vi "Stop.vi"(8 "error in (no error)":errorcluster, 10 "Message in":refnum<class "StopMessage.lvclass">, 11 "DAQCascade512II in":refnum<class "DAQCascade512II.lvclass">) -> (0 "error out":errorcluster, 3 "DAQCascade512II out":refnum<class "DAQCascade512II.lvclass">)   [LabVIEW 2012, in "DAQCascade512II.lvclass"]
doc: "This member function is called when the statemachine in the run.vi receives an 'stop' command. It relays the message to all observers of the component.\n\nOverride this member function in your derived class if you need additional stop functionality (but don't forget to call the parent method)."
uses:
  DAQCascade512II.lvclass
  <vilib>/Distrio/Murmex/StopMessage/StopMessage.lvclass
  <vilib>/Distrio/Murmex/Murmex/Murmex.lvclass
  DAQCascade512II.lvclass/DAQCascade512II.ctl
  <vilib>/Distrio/Murmex/TerminateMessage/TerminateMessage class.ctl
  <vilib>/Distrio/Murmex/TerminateMessage/TerminateMessage.lvclass
panel:
  # "This method is called when the STOP\ntrigger is sent. \n\nOverride this method when your component needs to\nrespond to this trigger. \n\nCall parent for proper implementation"
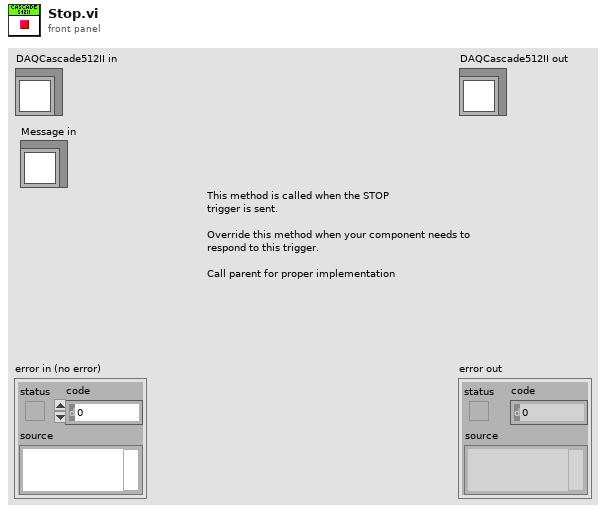
[diagram p1: front panel]
types:
  T1 = typedef "Murmex.lvlib/TerminateMessage.lvclass/TerminateMessage class.ctl" = refnum<class "TerminateMessage.lvclass">
  T2 = typedef "IMAQ Image.ctl" = refnum<image>
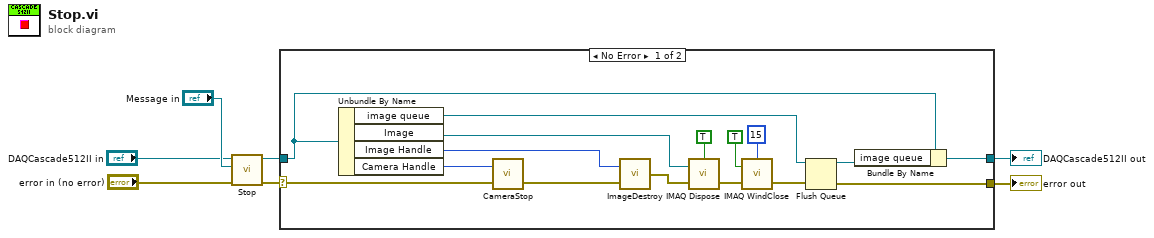
[diagram p0: block diagram]
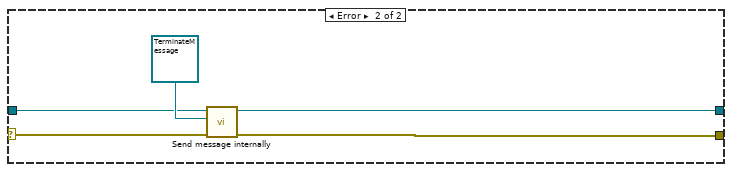
[diagram p2: hidden frame]
diagram:
  n1 = call-parent "Stop.vi"("error in (no error)"="error in (no error)", "Message in"="Message in", "Murmex in"="DAQCascade512II in") -> ("error out"=w6:errorcluster, "Murmex out"=w5:refnum<class "DAQCascade512II.lvclass">)  [unwired: 7 in]
  n2 = case shown="No Error" w6 {
    selector: w6 -> [w23 w25]
    tunnel: w5 -> [w10 w27]
    tunnel: [w8 w26] -> w4
    tunnel: [w12 w24] -> w3
    frame No Error {
      n3 = Unbundle By Name(w10) -> ("image queue"=w11:refnum<queue>, "Image"=w18:T2, "Image Handle"=w21:u32, "Camera Handle"=w22:u32)
      n4 = call <userlib>:"CameraStop.vi"("error in"=w23, "Camera Handle"=w22) -> ("error out"=w14:errorcluster)  [unwired: 1 out]
      n5 = call <userlib>:"ImageDestroy.vi"("error in"=w14, "Data handle"=w21) -> ("error out"=w20:errorcluster)
      n6 = call "IMAQ Dispose"("All Images? (No)"=TRUE, "Image"=w18, "error in (no error)"=w20) -> ("error out"=w15:errorcluster)  [unwired: 3 in]
      n7 = call "IMAQ WindClose"("Window Number (0...15)"=15, "Close All Windows (False)"=TRUE, "error in (no error)"=w15) -> ("error out"=w13:errorcluster)  [unwired: 3 in]
      n8 = Flush Queue(queue=w11, error in (no error)=w13) -> (queue out=w9:refnum<queue>, error out=w12:errorcluster)  [unwired: 1 out]
      n9 = Bundle By Name(cluster=w10, "image queue"=w9) -> (w8:refnum<class "DAQCascade512II.lvclass">)
    }
    frame Error {
      n10 = call <vilib>:"Send message internally.vi"("error in (no error)"=w25, "Message"=T1 refnum ("TerminateMessage.lvclass"), "Murmex in"=w27) -> ("error out"=w24:errorcluster, "Murmex out"=w26:refnum<class "DAQCascade512II.lvclass">)  [unwired: 7 in]
    }
  }
  "error out" <- w3
  "DAQCascade512II out" <- w4
